vi "Caterpillar.vi"   [LabVIEW 2012]
uses:
  <vilib>/Rock Robotics/WPI/Solenoid/WPI_SolenoidValue.ctl
  <vilib>/Rock Robotics/WPI/SafetyOutput/WPI_SafetyOutputConfigMenu.ctl
  Begin/Global Refnums.vi
  Begin/Global Variables.vi
  <vilib>/Rock Robotics/WPI/Solenoid/WPI_SolenoidSetEnum.vi
types:
  T1 = typedef "WPI_DigitalInputDevRef.ctl" = cluster{"DevStatus":errorcluster, "DIO Channel":T2, "Digital Module":T3}
  T2 = typedef "FPGA_DIOChannel.ctl" = enum8{"DIO 1", "DIO 2", "DIO 3", "DIO 4", "DIO 5", "DIO 6", "DIO 7", "DIO 8", "DIO 9", "DIO 10", "DIO 11", "DIO 12", "DIO 13", "DIO 14", "Invalid"}
  T3 = typedef "FPGA_TypedefDigitalModule.ctl" = enum16{"Digital Module 1", "Digital Module 2"}
  T4 = typedef "WPI_MotorControlDeviceRef.ctl" = cluster{"DeviceStatus":errorcluster, "Type":enum16{"PWM", "CAN"}, "PWM":cluster{"Digital Module":T3, "PWM Channel":T5, "DeadBand":T6}, "CAN":cluster{"Device Number":u8, "Control Mode":T7, "Semaphore":T8, "Max Vout":dbl}, "Invert":bool, "TransformRef":T9, "InvTransformRef":T9}
  T5 = typedef "FPGA_DIOPWMChannel.ctl" = enum8{"PWM 1", "PWM 2", "PWM 3", "PWM 4", "PWM 5", "PWM 6", "PWM 7", "PWM 8", "PWM 9", "PWM 10", "Invalid"}
  T6 = typedef "WPI_PWMDeadband.ctl" = cluster{"Name":string, "maxPositivePwm":i32, "minPositivePwm":i32, "centerPwm":i32, "maxNegativePwm":i32, "minNegativePwm":i32, "angularRange":u16}
  T7 = typedef "WPI_CANJaguar_ControlMode.ctl" = enum8{"Percent VBus", "Current", "Speed", "Position", "Voltage"}
  T8 = typedef "Semaphore RefNum" = refnum<k1>
  T9 = typedef "WPI_PWMTransform_ConPane.ctl" = refnum<vi>
  T10 = typedef "WPI_SolenoidValue.ctl" = enum16{"Off", "On", "Forward", "Reverse"}
  T11 = typedef "WPI_SafetyOutputConfigMenu.ctl" = enum16{"Enable", "Disable"}
  T12 = typedef "WPI_SolenoidDevRef.ctl" = cluster{"DevStatus":errorcluster, "Solenoid Module":T13, "Forward Solenoid Channel":T14, "Reverse Solenoid Channel":T14}
  T13 = typedef "FPGA_TypedefSolenoidModule.ctl" = enum16{"Solenoid Module 1", "Solenoid Module 2"}
  T14 = typedef "WPI_SolenoidChannel.ctl" = enum8{"Solenoid 1", "Solenoid 2", "Solenoid 3", "Solenoid 4", "Solenoid 5", "Solenoid 6", "Solenoid 7", "Solenoid 8", "Invalid"}
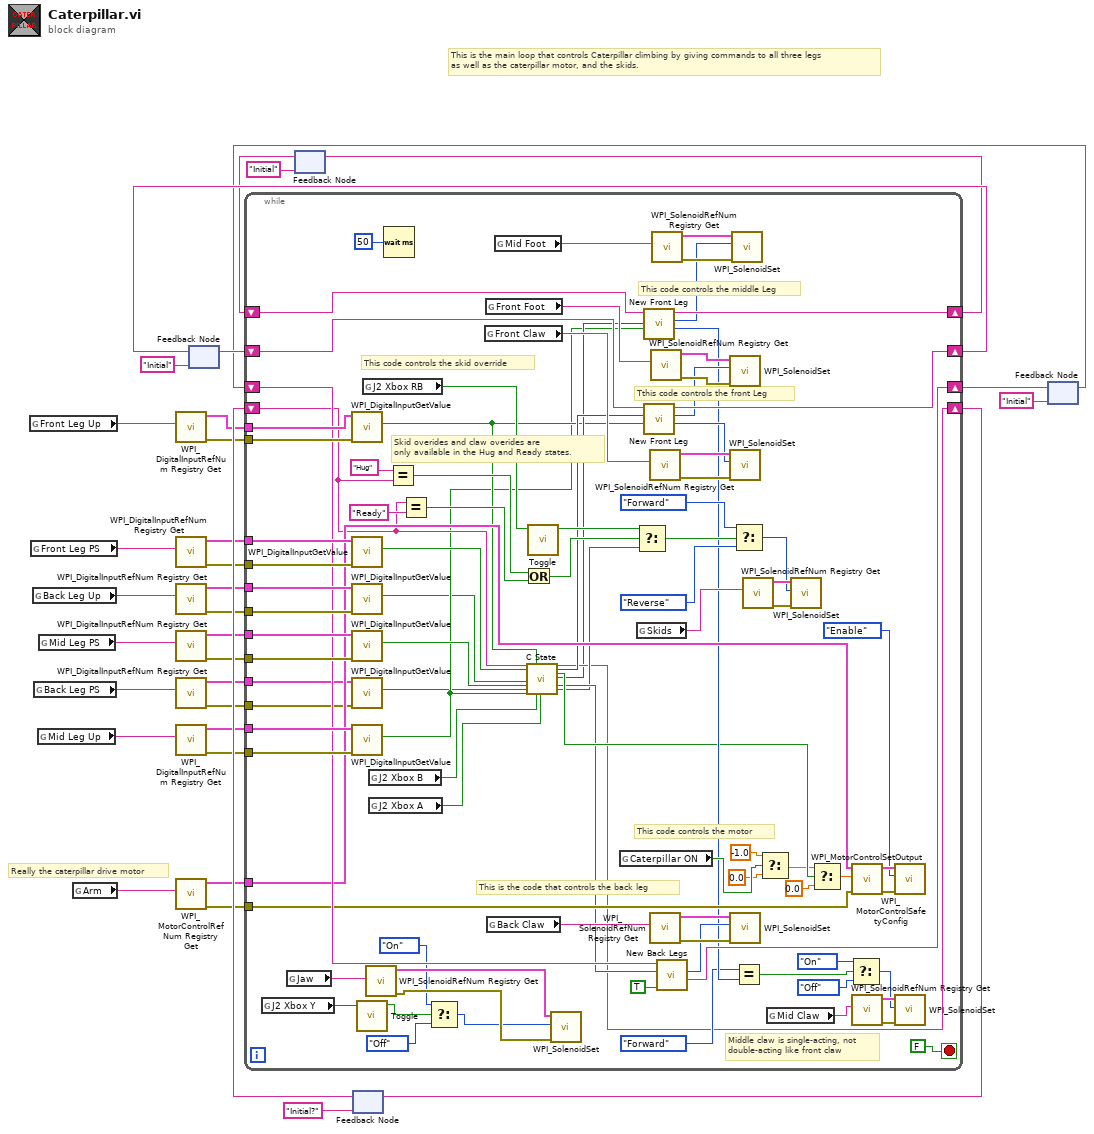
[diagram p0: block diagram]
diagram:
  # "This is the main loop that controls Caterpillar climbing by giving commands to all three legs\nas well as the caterpillar motor, and the skids."
  # "Really the caterpillar drive motor"
  n1 = global read "Global Refnums.vi" "Front Leg Up"() -> (w4:string)
  n2 = global read "Global Refnums.vi" "Front Leg PS"() -> (w7:string)
  n3 = global read "Global Refnums.vi" "Back Leg Up"() -> (w5:string)
  n4 = global read "Global Refnums.vi" "Back Leg PS"() -> (w3:string)
  n5 = global read "Global Refnums.vi" "Mid Leg Up"() -> (w6:string)
  n6 = global read "Global Refnums.vi" "Mid Leg PS"() -> (w8:string)
  n7 = global read "Global Refnums.vi" "Arm"() -> (w9:string)
  n8 = call <vilib>:"WPI_DigitalInputRefNum Registry Get.vi"("refnum name"=w4) -> ("error out"=w12:errorcluster, "DigitalInputDevRef"=w13:T1)  [unwired: 9 in]
  n9 = call <vilib>:"WPI_DigitalInputRefNum Registry Get.vi"("refnum name"=w7) -> ("error out"=w26:errorcluster, "DigitalInputDevRef"=w30:T1)  [unwired: 9 in]
  n10 = call <vilib>:"WPI_DigitalInputRefNum Registry Get.vi"("refnum name"=w5) -> ("error out"=w23:errorcluster, "DigitalInputDevRef"=w27:T1)  [unwired: 9 in]
  n11 = call <vilib>:"WPI_DigitalInputRefNum Registry Get.vi"("refnum name"=w8) -> ("error out"=w25:errorcluster, "DigitalInputDevRef"=w29:T1)  [unwired: 9 in]
  n12 = call <vilib>:"WPI_DigitalInputRefNum Registry Get.vi"("refnum name"=w3) -> ("error out"=w1:errorcluster, "DigitalInputDevRef"=w2:T1)  [unwired: 9 in]
  n13 = call <vilib>:"WPI_DigitalInputRefNum Registry Get.vi"("refnum name"=w6) -> ("error out"=w24:errorcluster, "DigitalInputDevRef"=w28:T1)  [unwired: 9 in]
  n14 = call <vilib>:"WPI_MotorControlRefNum Registry Get.vi"("refnum name"=w9) -> ("error out"=w10:errorcluster, "MotorControlDevRef"=w11:T4)  [unwired: 9 in]
  n15 = feedback #1("Initial" ("New state")) -> (w21:string)
  n16 = feedback #2("Initial" ("Old state")) -> (w15:string)
  n17 = feedback #3("Initial?" ("New State")) -> (w32:string)
  n18 = feedback #4("Initial" ("Old state")) -> (w18:string)
  n19 = while {
    shift-right: [w51] -> w33
    shift-left: w32 -> [w48]
    tunnel: w30 -> [w126]
    tunnel: w29 -> [w125]
    tunnel: w28 -> [w124]
    tunnel: w27 -> [w123]
    tunnel: w26 -> [w122]
    tunnel: w25 -> [w121]
    tunnel: w24 -> [w120]
    tunnel: w23 -> [w119]
    shift-right: [w110] -> w22
    shift-left: w21 -> [w100]
    shift-right: [w102] -> w19
    shift-left: w18 -> [w103]
    shift-right: [w74] -> w16
    shift-left: w15 -> [w75]
    tunnel: w13 -> [w109]
    tunnel: w12 -> [w108]
    tunnel: w11 -> [w98]
    tunnel: w10 -> [w97]
    tunnel: w2 -> [w69]
    tunnel: w1 -> [w68]
    stop <- FALSE stop-if-true
    # "Skid overides and claw overides are\nonly available in the Hug and Ready states."
    # "This code controls the motor"
    # "This is the code that controls the back leg"
    # "Middle claw is single-acting, not\ndouble-acting like front claw"
    # "Tthis code controls the front Leg"
    # "This code controls the middle Leg"
    # "This code controls the skid override"
    n20 = global read "Global Variables.vi" "J2 Xbox Y"() -> (w41:bool)
    n21 = global read "Global Refnums.vi" "Jaw"() -> (w40:string)
    n22 = call <vilib>:"WPI_DigitalInputGetValue.vi"("error in (no error)"=w108, "DigitalInputDevRef"=w109) -> ("Value"=w49:bool)  [unwired: 7 in, 2 out]
    n23 = call <vilib>:"WPI_DigitalInputGetValue.vi"("error in (no error)"=w122, "DigitalInputDevRef"=w126) -> ("Value"=w47:bool)  [unwired: 7 in, 2 out]
    n24 = call <vilib>:"WPI_DigitalInputGetValue.vi"("error in (no error)"=w119, "DigitalInputDevRef"=w123) -> ("Value"=w43:bool)  [unwired: 7 in, 2 out]
    n25 = call <vilib>:"WPI_DigitalInputGetValue.vi"("error in (no error)"=w121, "DigitalInputDevRef"=w125) -> ("Value"=w46:bool)  [unwired: 7 in, 2 out]
    n26 = call <vilib>:"WPI_DigitalInputGetValue.vi"("error in (no error)"=w68, "DigitalInputDevRef"=w69) -> ("Value"=w44:bool)  [unwired: 7 in, 2 out]
    n27 = call <vilib>:"WPI_DigitalInputGetValue.vi"("error in (no error)"=w120, "DigitalInputDevRef"=w124) -> ("Value"=w45:bool)  [unwired: 7 in, 2 out]
    n28 = call "Toggle.vi"("Boolean"=w41) -> ("Toggled"=w34:bool)  [unwired: 10 in]
    n29 = global read "Global Variables.vi" "J2 Xbox RB"() -> (w80:bool)
    n30 = call <vilib>:"WPI_SolenoidRefNum Registry Get.vi"("refnum name"=w40) -> ("error out"=w38:errorcluster, "SolenoidDevRef"=w39:T12)  [unwired: 9 in]
    n31 = global read "Global Variables.vi" "J2 Xbox B"() -> (w56:bool)
    n32 = global read "Global Variables.vi" "J2 Xbox A"() -> (w57:bool)
    n33 = Wait (ms)(milliseconds to wait=u32 50) -> ()  [unwired: 1 out]
    n34 = Equal?(x="Hug", y=w48) -> (x = y?=w85:bool)
    n35 = Equal?(x=w48, y="Ready") -> (x = y?=w87:bool)
    n36 = Select(t=WPI_SolenoidValue."On" ("Foot"), s=w34, f=WPI_SolenoidValue."Off" ("Foot")) -> (s? t:f=w35:T10)
    n37 = global read "Global Refnums.vi" "Front Claw"() -> (w93:string)
    n38 = global read "Global Refnums.vi" "Front Foot"() -> (w94:string)
    n39 = global read "Global Refnums.vi" "Back Claw"() -> (w92:string)
    n40 = global read "Global Refnums.vi" "Mid Foot"() -> (w71:string)
    n41 = Or(x=w85, y=w87) -> (x .or. y?=w78:bool)
    n42 = call "C State.vi"("State"=w48, "Front Leg PS"=w47, "Back Leg Up"=w43, "Mid Leg PS"=w46, "Back Leg PS"=w44, "Mid Leg Up"=w45, "Front Leg Up"=w49, "Back Claws Cmd"=w56, "Front Claw Cmd"=w57) -> ("newState"=w51:string, "Front Leg Cmd"=w55:enum16{"Down Closed", "Down Opened", "Up"}, "Drive Motor Enabled"=w54:bool, "Mid Leg Cmd"=w50:enum16{"Down Closed", "Down Opened", "Up"}, "Engage Back Leg"=w53:bool, "Skids"=w52:bool)  [unwired: 13 in]
    n43 = call "Toggle.vi"("Boolean"=w80) -> ("Toggled"=w77:bool)  [unwired: 10 in]
    n44 = call-poly <vilib>:"WPI_SolenoidSet.vi"("error in (no error)"=w38, "Value"=w35, "SolenoidDevRef"=w39) -> ()  [unwired: 7 in, 2 out]
    n45 = global read "Global Variables.vi" "Caterpillar ON"() -> (w67:bool)
    n46 = Select(t=w77, s=w78, f=w52) -> (s? t:f=w76:bool)
    n47 = global read "Global Refnums.vi" "Skids"() -> (w91:string)
    n48 = call "New Front Leg.vi"("Leg up"=w45, "Command"=w50, "Old State"=w75) -> ("Claw"=w65:T10, "Foot"=w70:T10, "New state"=w74:string)  [unwired: 6 in]
    n49 = call "New Front Leg.vi"("Leg up"=w49, "Command"=w55, "Old State"=w100) -> ("Claw"=w83:T10, "Foot"=w81:T10, "New state"=w110:string)  [unwired: 6 in]
    n50 = call <vilib>:"WPI_SolenoidRefNum Registry Get.vi"("refnum name"=w93) -> ("error out"=w116:errorcluster, "SolenoidDevRef"=w115:T12)  [unwired: 9 in]
    n51 = call <vilib>:"WPI_SolenoidRefNum Registry Get.vi"("refnum name"=w92) -> ("error out"=w112:errorcluster, "SolenoidDevRef"=w111:T12)  [unwired: 9 in]
    n52 = call <vilib>:"WPI_SolenoidRefNum Registry Get.vi"("refnum name"=w94) -> ("error out"=w118:errorcluster, "SolenoidDevRef"=w117:T12)  [unwired: 9 in]
    n53 = call <vilib>:"WPI_SolenoidRefNum Registry Get.vi"("refnum name"=w71) -> ("error out"=w73:errorcluster, "SolenoidDevRef"=w72:T12)  [unwired: 9 in]
    n54 = call "New Back Legs.vi"("isDualActing"=TRUE, "Engage Leg 1/2"=w53, "New state"=w103) -> ("Old state"=w102:string, "Claw"=w82:T10)  [unwired: 7 in]
    n55 = call-poly <vilib>:"WPI_SolenoidSet.vi"("error in (no error)"=w118, "Value"=w81, "SolenoidDevRef"=w117) -> ()  [unwired: 7 in, 2 out]
    n56 = call-poly <vilib>:"WPI_SolenoidSet.vi"("error in (no error)"=w116, "Value"=w83, "SolenoidDevRef"=w115) -> ()  [unwired: 7 in, 2 out]
    n57 = call-poly <vilib>:"WPI_SolenoidSet.vi"("error in (no error)"=w112, "Value"=w82, "SolenoidDevRef"=w111) -> ()  [unwired: 7 in, 2 out]
    n58 = call-poly <vilib>:"WPI_SolenoidSet.vi"("error in (no error)"=w73, "Value"=w70, "SolenoidDevRef"=w72) -> ()  [unwired: 7 in, 2 out]
    n59 = Select(t=WPI_SolenoidValue."Forward" ("Value"), s=w76, f=WPI_SolenoidValue."Reverse" ("Value")) -> (s? t:f=w79:T10)
    n60 = Equal?(x=WPI_SolenoidValue."Forward" ("Value"), y=w65) -> (x = y?=w66:bool)
    n61 = call <vilib>:"WPI_SolenoidRefNum Registry Get.vi"("refnum name"=w91) -> ("error out"=w107:errorcluster, "SolenoidDevRef"=w106:T12)  [unwired: 9 in]
    n62 = Select(t=-1.0, s=w67, f=0.0) -> (s? t:f=w42:dbl)
    n63 = global read "Global Refnums.vi" "Mid Claw"() -> (w95:string)
    n64 = call-poly <vilib>:"WPI_SolenoidSet.vi"("error in (no error)"=w107, "Value"=w79, "SolenoidDevRef"=w106) -> ()  [unwired: 7 in, 2 out]
    n65 = Select(t=w42, s=w54, f=0.0) -> (s? t:f=w58:dbl)
    n66 = Select(t=WPI_SolenoidValue."On" ("Value"), s=w66, f=WPI_SolenoidValue."Off" ("Value")) -> (s? t:f=w61:T10)
    n67 = call <vilib>:"WPI_MotorControlSetOutput.vi"("error in (no error)"=w97, "Output"=w58, "MotorControlDevRef"=w98) -> ("error out"=w89:errorcluster, "MotorControlDevRef"=w90:T4)  [unwired: 6 in, 1 out]
    n68 = call <vilib>:"WPI_SolenoidRefNum Registry Get.vi"("refnum name"=w95) -> ("error out"=w114:errorcluster, "SolenoidDevRef"=w113:T12)  [unwired: 9 in]
    n69 = call <vilib>:"WPI_MotorControlSafetyConfig.vi"("error in (no error)"=w89, "mode"=WPI_SafetyOutputConfigMenu."Enable", "MotorControlDevRef"=w90) -> ()  [unwired: 7 in, 2 out]
    n70 = call-poly <vilib>:"WPI_SolenoidSet.vi"("error in (no error)"=w114, "Value"=w61, "SolenoidDevRef"=w113) -> ()  [unwired: 7 in, 2 out]
  }
  n71 = feedback-in #1(w22) -> ()
  n72 = feedback-in #2(w16) -> ()
  n73 = feedback-in #3(w33) -> ()
  n74 = feedback-in #4(w19) -> ()
